vi "FreeUnpackedFields.vi"(8 "error in":errorcluster, 11 "Unpacked Fields ID":T1) -> (0 "error out":errorcluster)   [LabVIEW 2019, in "gprc-lvsupport.lvlib"]
uses:
  gprc-lvsupport.lvlib
  Shared/grpcId.ctl
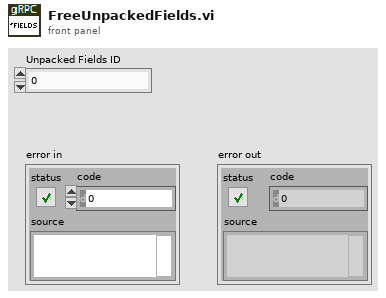
[diagram p1: front panel]
types:
  T1 = typedef "gprc-lvsupport.lvlib/grpcId.ctl" = u64
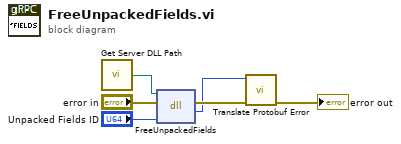
[diagram p0: block diagram]
diagram:
  n1 = call "Get Server DLL Path.vi"() -> ("Server dll path"=w4:path)
  n2 = dll-call lib="?" fn="FreeUnpackedFields"(path in=w4, error in="error in", "serializationId"="Unpacked Fields ID") -> (error out=w5:errorcluster, "return type"=w1:i32)  [unwired: 2 in, 1 out]
  n3 = call "Translate Protobuf Error.vi"("error in"=w5, "Error Code"=w1) -> ("error out"=→"error out":errorcluster)  [unwired: 9 in]
